vi "FormatAuthorizationString.vi"(7 "password":string, 9 "ServerInfo":T1, 10 "String in":string, 11 "Username":string) -> (3 "String out":string)   [LabVIEW 2016]
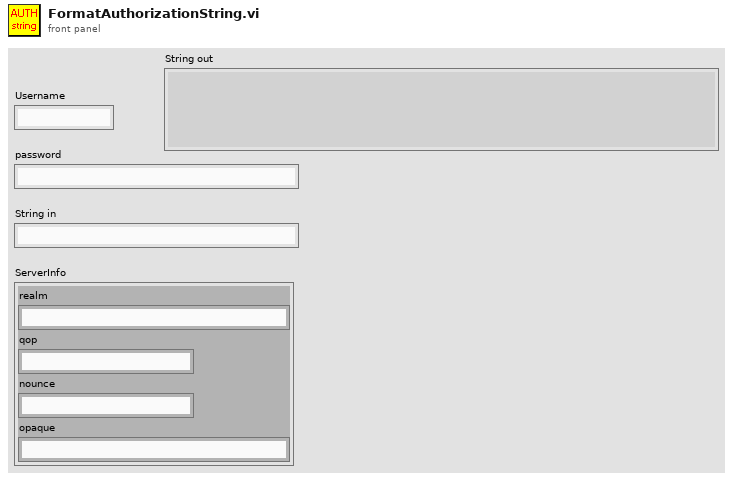
[diagram p1: front panel]
types:
  T1 = cluster{"realm":string, "qop":string, "nounce":string, "opaque":string}
  T2 = cluster{"nonce from server":string, "qop ":string}
  T3 = cluster{"username":string, "realm":string, "password":string, "method":string, "digestURI":string}
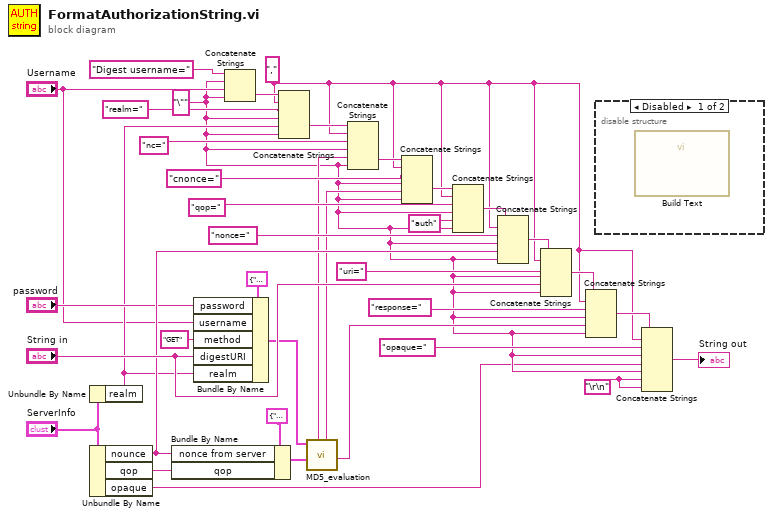
[diagram p0: block diagram]
diagram:
  w3 = "\r\n"
  w1 = "," ("string")
  w6 = "\"" ("string")
  n1 = Unbundle By Name("ServerInfo") -> ("realm"=w18:string)
  n2 = Unbundle By Name("ServerInfo") -> ("nounce"=w32:string, "qop"=w8:string, "opaque"=w5:string)
  n3 = Bundle By Name(cluster=T2 {"nonce from server"="ÜÙ‹q\u0002Ý/\u000e‹\u0011Ðö\u0000¿°À“", "qop "="auth"} ("ServerInfo"), "nonce from server"=w32, "qop"=w8) -> (w22:T2)
  n4 = Bundle By Name(cluster=T3 {"username"="Mufasa", "realm"="testrealm@host.com", "password"="Circle Of Life", "method"="GET", "digestURI"="/dir/index.html"} ("ClientInfo"), "password"="password", "username"="Username", "method"="GET", "digestURI"="String in", "realm"=w18) -> (w20:T3)
  n5 = Concatenate Strings("Digest username=", w6, "Username", w6) -> (w10:string)
  n6 = Concatenate Strings(w10, w1, "realm=", w6, w18, w6) -> (w14:string)
  n7 = call "MD5_evaluation.vi"("ServerInfo"=w22, "ClientInfo"=w20) -> ("response"=w38:string, "cnonce of client"=w26:string, "RequestCounter"=w23:string)  [unwired: 5 in, 2 out]
  n8 = Concatenate Strings(w14, w1, "nc=", w6, w23, w6) -> (w24:string)
  n9 = Concatenate Strings(w24, w1, "cnonce=", w6, w26, w6) -> (w27:string)
  n10 = Concatenate Strings(w27, w1, "qop=", w6, "auth" ("string"), w6) -> (w30:string)
  n11 = Concatenate Strings(w30, w1, "nonce=", w6, w32, w6) -> (w33:string)
  n12 = Concatenate Strings(w33, w1, "uri=", w6, "String in", w6) -> (w36:string)
  n13 = Concatenate Strings(w36, w1, "response=", w6, w38, w6) -> (w2:string)
  n14 = disable-structure shown="Disabled" {
    frame Disabled {
      n15 = call "Build Text"() -> ()  [unwired: 14 in, 2 out]
    }
    frame Enabled {
    }
  }
  n16 = Concatenate Strings(w2, w1, "opaque=", w6, w5, w6, w3, w3) -> (→"String out":string)
